vi "CPU Temperature.vi"(8 "error in (no error)":errorcluster, 11 "RP Instrument in":refnum<class "RP Instrument.lvclass">) -> (0 "error out":errorcluster, 2 "CPU Temperature":dbl, 3 "RP Instrument out":refnum<class "RP Instrument.lvclass">)   [LabVIEW 2016, in "RP Instrument.lvclass"]
uses:
  RP Instrument.lvclass
  RP Instrument.lvclass/RP Instrument.ctl
  RP Communicator/RP Communicator.lvclass
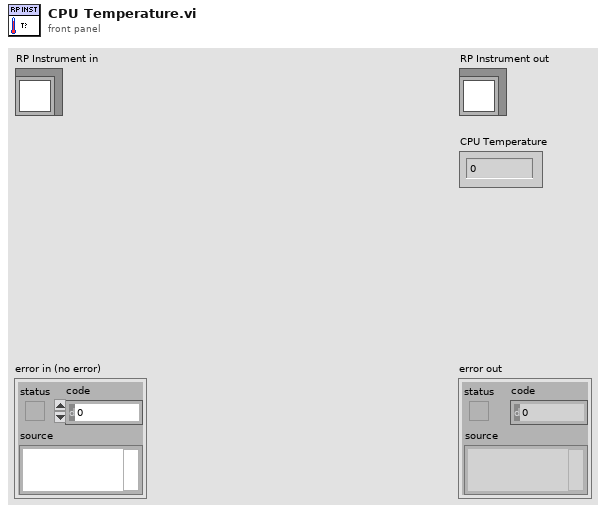
[diagram p1: front panel]
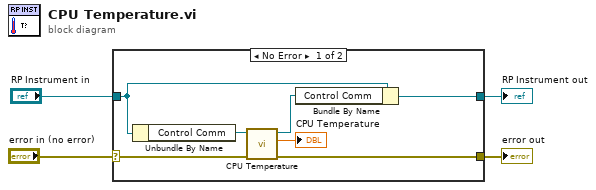
[diagram p0: block diagram]
diagram:
  n1 = case shown="No Error" "error in (no error)" {
    selector: "error in (no error)" -> [w6 w13]
    tunnel: [w5 w13] -> w3
    tunnel: [w8 w12] -> w1
    tunnel: "RP Instrument in" -> [w11 w12]
    frame No Error {
      n2 = Unbundle By Name(w11) -> ("Control Comm"=w10:refnum<class "RP Communicator.lvclass">)
      n3 = call-dynamic "CPU Temperature.vi"("error in (no error)"=w6, "RP Communicator in"=w10) -> ("error out"=w5:errorcluster, "CPU Temperature"=→"CPU Temperature":dbl, "RP Communicator out"=w7:refnum<class "RP Communicator.lvclass">)  [unwired: 7 in]
      n4 = Bundle By Name(cluster=w11, "Control Comm"=w7) -> (w8:refnum<class "RP Instrument.lvclass">)
    }
    frame Error {
    }
  }
  "error out" <- w3
  "RP Instrument out" <- w1
